vi "Write FPGA Session.vi"(8 "error in (no error)":errorcluster, 10 "FPGA Session":refnum<data-value>, 11 "gController in":refnum<class "gController.lvclass">) -> (0 "error out":errorcluster, 3 "gController out":refnum<class "gController.lvclass">)   [LabVIEW 2017, in "Controller.lvlib" / "gController.lvclass"]
uses:
  gController.lvclass
  Session/Raw FPGA/FPGA Session.lvclass
  C:/Program Files (x86)/National Instruments/LabVIEW 2017/vi.lib/MSR Consulting, LLC/General Reuse/Session APIs/_Session Fwk/Session - Root.lvclass
  gController.lvclass/gController.ctl
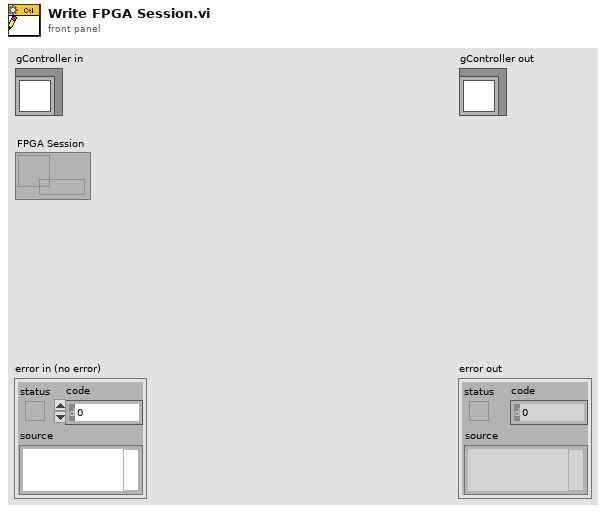
[diagram p1: front panel]
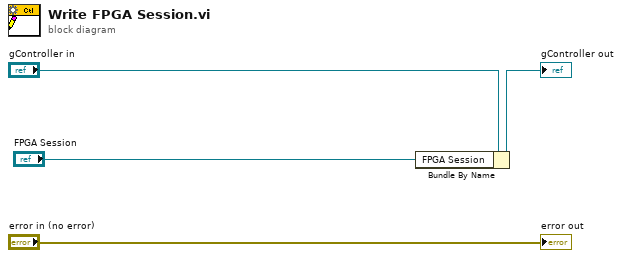
[diagram p0: block diagram]
diagram:
  n1 = Bundle By Name(cluster="gController in", "FPGA Session"="FPGA Session") -> (→"gController out":refnum<class "gController.lvclass">)
  "error out" <- "error in (no error)"
